vi "G#Object_SetError.vi"(0 "reference in":refnum<class "G#Object.lvclass">, 1 "error (F)":bool, 2 "source":string, 3 "code":i32=400040, 5 "error in (no error)":errorcluster, 6 "call depth (1)":i32=1) -> (19 "error out":errorcluster)   [LabVIEW 2020, in "G#Object.lvclass"]
doc: "Sets VI error."
uses:
  <vilib>/addons/_AddQ/G#Object/G#Object.lvclass
  <vilib>/addons/_AddQ/G#Object/utils/G#Object_EventType.ctl
  <vilib>/addons/_AddQ/G#Object/utils/G#Object_ObjectInfoType.ctl
  <vilib>/addons/_AddQ/G#Object/utils/G#Object_CreateMethod.ctl
  <vilib>/addons/_AddQ/G#Object/G#Object.lvclass/G#Object.ctl
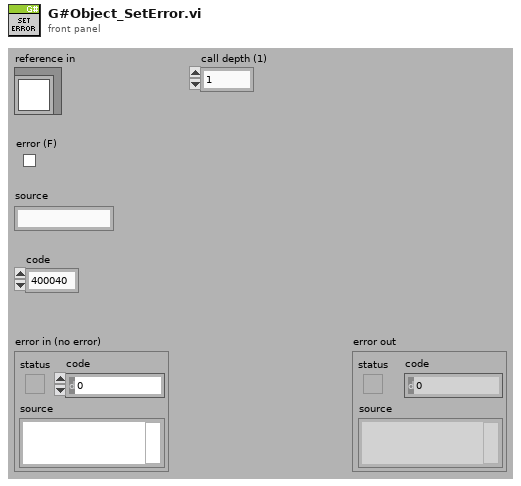
[diagram p1: front panel]
types:
  T1 = typedef "G#Object.lvclass/G#Object_ObjectInfoType.ctl" = cluster{"ObjectName":string, "ObjectID":u32, "Users":i32, "Counter":bool, "AttributeRefs":u32[], "FullClassName":string, "ClassName":string, "CreateMethod":T2, "GenericDestructorExists":bool, "Owner":string}
  T2 = typedef "G#Object.lvclass/G#Object_CreateMethod.ctl" = enum16{"Create", "Create or look up existing", "Look up existing"}
  T3 = typedef "G#Object.lvclass/G#Object_EventType.ctl" = enum16{"Created new", "Looked up existing", "Deleted", "Forced delete", "Not deleted", "Garbage collected", "Cleared", "User", "Error", "External create object", "External create class attributes", "Created class attributes", "Run constructor", "Run constructor done", "Run open method", "Run open method done"}
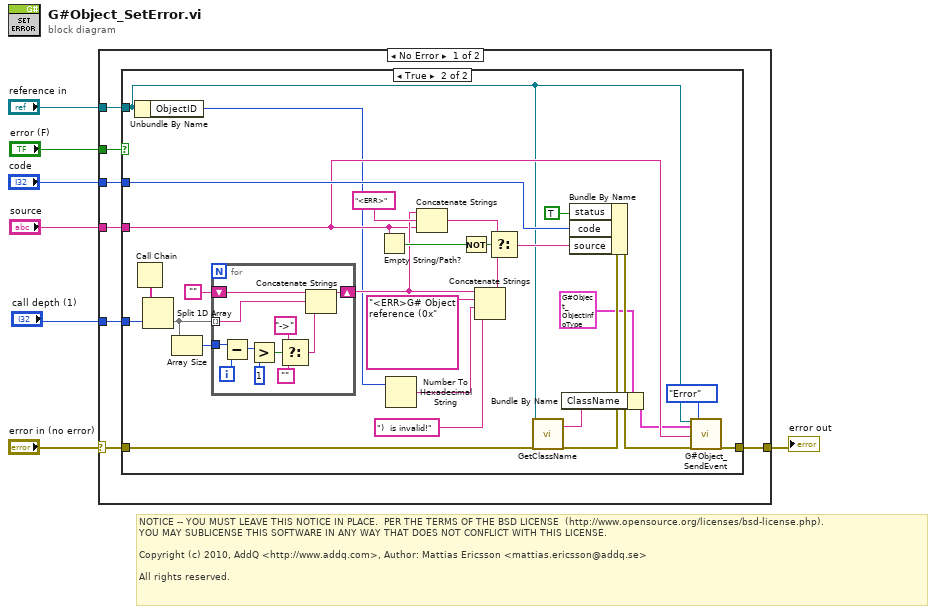
[diagram p0: block diagram]
diagram:
  # "NOTICE -- YOU MUST LEAVE THIS NOTICE IN PLACE.  PER THE TERMS OF THE BSD LICENSE  (http://www.opensource.org/licenses/bsd-license.php).\nYOU MAY SUBLICENSE THIS SOFTWARE IN ANY WAY THAT DOES NOT CONFLICT WITH THIS LICENSE.\n\nCopyright (c) 2010, AddQ <http://www.addq.com>, Author: Mattias Ericsson <mattias.ericsson@addq.se>\n\nAll rights reserved."
  n1 = case shown="No Error" "error in (no error)" {
    selector: "error in (no error)" -> [w13 w55]
    tunnel: [w9 w55] -> w1
    tunnel: "error (F)" -> [w14 _]
    tunnel: "source" -> [w12 _]
    tunnel: "call depth (1)" -> [w11 _]
    tunnel: "code" -> [w10 _]
    tunnel: "reference in" -> [w8 _]
    frame No Error {
      n2 = case shown="True" w14 {
        tunnel: w13 -> [w15 w21]
        tunnel: w12 -> [_ w23]
        tunnel: w11 -> [_ w30]
        tunnel: w10 -> [_ w29]
        tunnel: [w15 w26] -> w9
        tunnel: w8 -> [_ w19]
        frame False {
        }
        frame True {
          n3 = Unbundle By Name(w19) -> ("ObjectID"=w22:u32)
          n4 = Call Chain() -> (call chain=w43:string[])
          n5 = Split 1D Array(array=w43, index=w30) -> (second subarray=w42:string[])  [unwired: 1 out]
          n6 = Array Size(array=w42) -> (size(s)=w41:i32)
          n7 = for {
            shift-right: [w48] -> w28
            shift-left: "" -> [w50]
            tunnel: w42 -> [w49] mode=indexing
            tunnel: w41 -> [w54]
            i -> [w53]
            n8 = Subtract(x=w54, y=w53) -> (x-y=w52:i32)
            n9 = Greater?(x=w52, y=1) -> (0:w45:bool)
            n10 = Select(t="->", s=w45, f="") -> (s? t:f=w44:string)
            n11 = Concatenate Strings(w50, w49, w44) -> (w48:string)
          }
          n12 = Empty String/Path?(string/path=w23) -> (empty?=w33:bool)
          n13 = Number To Hexadecimal String(2:w22) -> (0:w38:string)  [unwired: 1 in]
          n14 = Concatenate Strings(w28, "<ERR>" ("Substring"), w23) -> (w32:string)
          n15 = Not(x=w33) -> (.not. x?=w34:bool)
          n16 = Concatenate Strings(w28, "<ERR>G# Object reference (0x" ("Substring"), w38, ")  is invalid!") -> (w35:string)
          n17 = Select(t=w32, s=w34, f=w35) -> (s? t:f=w27:string)
          n18 = call-dynamic "GetClassName.vi"("reference in"=w19, "error in (no error)"=w21) -> ("class name"=w17:string, "error out"=w20:errorcluster)  [unwired: 13 in, 3 out]
          n19 = Bundle By Name(cluster=T1 {"ObjectName"="", "ObjectID"=0, "Users"=0, "Counter"=FALSE, "AttributeRefs"=[], "FullClassName"="", "ClassName"="", "CreateMethod"=enum."Create", "GenericDestructorExists"=FALSE, "Owner"=""} ("object info extended"), "ClassName"=w17) -> (w16:T1)
          n20 = Bundle By Name(cluster=w20, "status"=TRUE ("Bundle Element"), "code"=w29, "source"=w27) -> (w25:errorcluster)
          n21 = call <vilib>:"G#Object_SendEvent.vi"("reference in"=w19, "object info extended"=w16, "comment"=w23, "error in (no error)"=w25, "G# event type"=G#Object_EventType."Error" ("G#Event")) -> ("error out"=w26:errorcluster)  [unwired: 14 in]
        }
      }
    }
    frame Error {
    }
  }
  "error out" <- w1
